vi "I2C Lidar Present.vi"(8 "error in (no error)":errorcluster, 11 "I2CDevRef":T1 {"Device Address" format="%.0x"}) -> (3 "Sensor Present":bool)   [LabVIEW 2014]
uses:
  <vilib>/Rock Robotics/WPI/I2C/WPI_I2CDevRef.ctl
  <vilib>/Rock Robotics/SystemInterfaces/Typedef/FPGA_TypedefDigitalModule.ctl
  <vilib>/Rock Robotics/SystemInterfaces/i2clib/i2c_bus.ctl
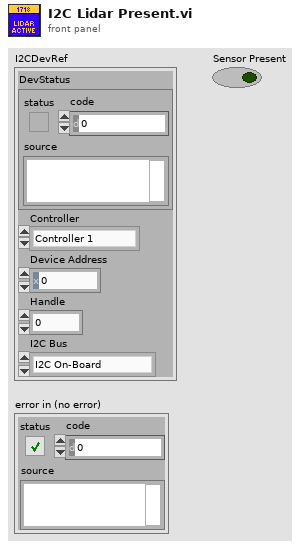
[diagram p1: front panel]
types:
  T1 = typedef "WPI_I2CDevRef.ctl" = cluster{"DevStatus":errorcluster, "Controller":T2, "Device Address":u8, "Handle":i32, "I2C Bus":T3}
  T2 = typedef "FPGA_TypedefDigitalModule.ctl" = enum16{"Controller 1"}
  T3 = typedef "i2c_bus.ctl" = enum16{"I2C On-Board", "I2C MXP", "Invalid"}
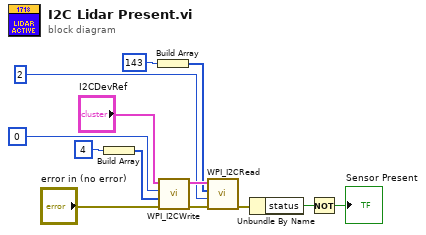
[diagram p0: block diagram]
diagram:
  n1 = Build Array(u8 4 ("Data To Send")) -> (w7:u8[])
  n2 = Build Array(u8 143 ("I2CRegister")) -> (w5:u8[])
  n3 = call <vilib>:"WPI_I2CWrite.vi"("error in (no error)"="error in (no error)", "I2CDataToSend"=w7, "I2CRegister"=u8 0 ("Data To Send"), "I2CDevRef"="I2CDevRef") -> ("error out"=w12:errorcluster, "I2CDevRef"=w6:T1)  [unwired: 6 out]
  n4 = call <vilib>:"WPI_I2CRead.vi"("error in (no error)"=w12, "I2CBytesToRead"=u8 2, "I2CRegister"=w5, "I2CDevRef"=w6) -> ("error out"=w13:errorcluster)  [unwired: 5 in, 2 out]
  n5 = Unbundle By Name(w13) -> ("status"=w2:bool)
  n6 = Not(x=w2) -> (.not. x?=→"Sensor Present":bool)
